vi "ep_Parameter Calculation.vi"(7 "reset? (F)":bool, 8 "error in (no error)":errorcluster, 9 "filter for frequency measurement":T2={"enable filter? (T)"=TRUE, "passband edge frequency [Hz]"=0.0, "passband ripple [dB]"=0.1, "stopband edge frequency [Hz]"=0.0, "stopband attenuation [dB]"=60.0}, 10 "frequency range [Hz]":cluster{"minimum":dbl, "maximum":dbl}, 11 "reference signal":waveform(dbl)) -> (0 "error out":errorcluster, 1 "total group delay [s]":dbl, 2 "parameters":T1, 3 "data out":dbl[](array[numeric]))   [LabVIEW 2013, in "NI_EP_Power Measurement.lvlib"]
uses:
  <vilib>/addons/Electrical Power/Power Measurement/NI_EP_Power Measurement.lvlib
  <vilib>/addons/Electrical Power/Power Measurement/subVIs/ep_Filter Design.ctl
  <vilib>/addons/Electrical Power/PQ/Resampling/Desktop/subVIs/ep_Parameters.ctl
  <vilib>/addons/Electrical Power/PQ/Resampling/NI_EP_Resample_Host.lvlib
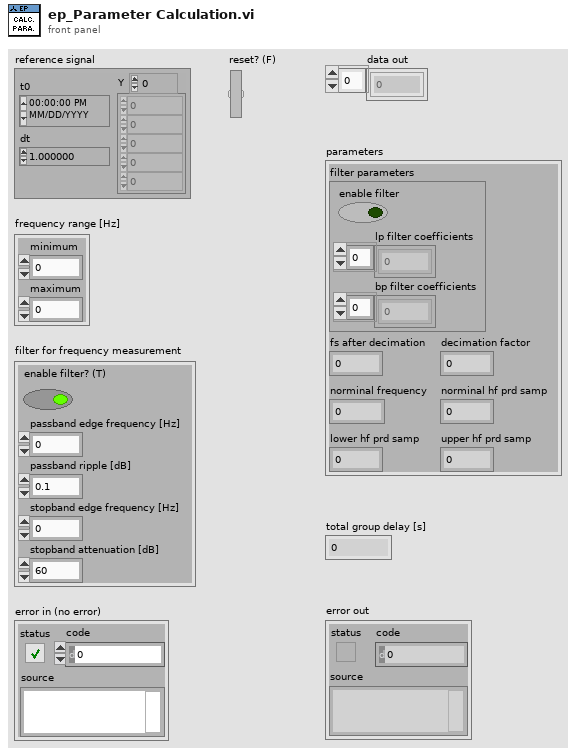
[diagram p1: front panel]
types:
  T1 = typedef "NI_EP_Resample_Host.lvlib/ep_Parameters.ctl" = cluster{"filter parameters":cluster{"enable filter":bool, "lp filter coefficients":dbl[], "bp filter coefficients":dbl[]}, "fs after decimation":dbl, "decimation factor":i32, "norminal frequency":dbl, "norminal hf prd samp":dbl, "lower hf prd samp":i32, "upper hf prd samp":i32}
  T2 = typedef "NI_EP_Power Measurement.lvlib/ep_Filter Design.ctl" = cluster{"enable filter? (T)":bool, "passband edge frequency [Hz]":dbl, "passband ripple [dB]":dbl, "stopband edge frequency [Hz]":dbl, "stopband attenuation [dB]":dbl}
  T3 = cluster{"enable filter":bool, "lp filter coefficients":dbl[], "bp filter coefficients":dbl[]}
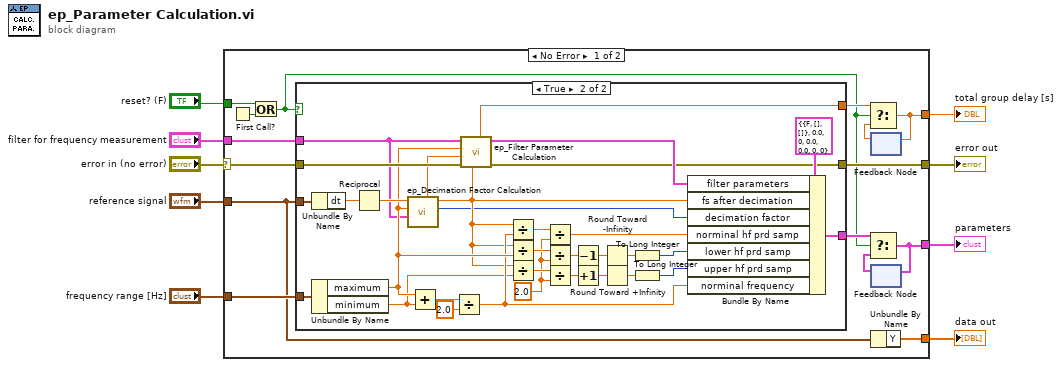
[diagram p0: block diagram]
diagram:
  n1 = case shown="No Error" "error in (no error)" {
    selector: "error in (no error)" -> [w20 w58]
    tunnel: "reset? (F)" -> [w23 _]
    tunnel: "reference signal" -> [w11 _]
    tunnel: "filter for frequency measurement" -> [w22 _]
    tunnel: "frequency range [Hz]" -> [w21 _]
    tunnel: [w19 w58] -> w5
    tunnel: [w16 _] -> w4
    tunnel: [w13 _] -> w3
    tunnel: [w10 _] -> w1
    frame No Error {
      n2 = First Call?() -> (First Call?: T/F=w24:bool)
      n3 = Or(x=w23, y=w24) -> (x .or. y?=w12:bool)
      n4 = case shown="True" w12 {
        tunnel: w11 -> [_ w57]
        tunnel: w22 -> [_ w26]
        tunnel: w21 -> [_ w54]
        tunnel: w20 -> [w25 w50]
        tunnel: [w25 w44] -> w19
        tunnel: [_ w34] -> w15
        tunnel: [_ w45] -> w17
        frame False {
        }
        frame True {
          w35 = 2.0 ("y")
          n5 = Unbundle By Name(w57) -> ("dt"=w56:dbl)
          n6 = Unbundle By Name(w54) -> ("maximum"=w48:dbl, "minimum"=w31:dbl)
          n7 = Reciprocal(x=w56) -> (1/x=w51:dbl)
          n8 = call <vilib>:"ep_Decimation Factor Calculation.vi"("filter for frequency measurement"=w26, "maximum frequency [Hz]"=w48, "fs [Hz]"=w51) -> ("decimation factor"=w28:i32, "fs after decimation [Hz]"=w29:dbl, "dup fs [Hz]"=w30:dbl)  [unwired: 6 in]
          n9 = Add(x=w48, y=w31) -> (x+y=w53:dbl)
          n10 = Divide(x=w53, y=2.0) -> (x/y=w43:dbl)
          n11 = call <vilib>:"ep_Filter Parameter Calculation.vi"("fs after decimation [Hz]"=w29, "error in (no error)"=w50, "fs [Hz]"=w30, "maximum frequency [Hz]"=w48, "filter for frequency measurement"=w26) -> ("error out"=w44:errorcluster, "filter parameters"=w49:T3, "total group delay [s]"=w34:dbl)  [unwired: 4 in]
          n12 = Divide(x=w29, y=w43) -> (x/y=w41:dbl)
          n13 = Divide(x=w29, y=w48) -> (x/y=w40:dbl)
          n14 = Divide(x=w29, y=w31) -> (x/y=w39:dbl)
          n15 = Divide(x=w41, y=w35) -> (x/y=w36:dbl)
          n16 = Divide(x=w40, y=w35) -> (x/y=w37:dbl)
          n17 = Divide(x=w39, y=w35) -> (x/y=w38:dbl)
          n18 = Decrement(x=w37) -> (x-1=w33:dbl)
          n19 = Increment(x=w38) -> (x+1=w32:dbl)
          n20 = Round Toward -Infinity(1:w33) -> (0:w47:dbl)
          n21 = Round Toward +Infinity(x=w32) -> (ceil(x): smallest int >= x=w46:dbl)
          n22 = To Long Integer(number=w47) -> (32bit integer=w42:i32)
          n23 = To Long Integer(number=w46) -> (32bit integer=w27:i32)
          n24 = Bundle By Name(cluster=T1 {"filter parameters"={"enable filter"=FALSE, "lp filter coefficients"=[], "bp filter coefficients"=[]}, "fs after decimation"=0.0, "decimation factor"=0, "norminal frequency"=0.0, "norminal hf prd samp"=0.0, "lower hf prd samp"=0, "upper hf prd samp"=0} ("output cluster 2"), "filter parameters"=w49, "fs after decimation"=w29, "decimation factor"=w28, "norminal hf prd samp"=w36, "lower hf prd samp"=w42, "upper hf prd samp"=w27, "norminal frequency"=w43) -> (w45:T1)
        }
      }
      n25 = feedback #1() -> (w14:dbl)  [unwired: 1 in]
      n26 = Select(t=w15, s=w12, f=w14) -> (s? t:f=w13:dbl)
      n27 = feedback-in #1(w13) -> ()
      n28 = feedback #2() -> (w18:T1)  [unwired: 1 in]
      n29 = Select(t=w17, s=w12, f=w18) -> (s? t:f=w16:T1)
      n30 = feedback-in #2(w16) -> ()
      n31 = Unbundle By Name(w11) -> ("Y"=w10:dbl[])
    }
    frame Error {
    }
  }
  "error out" <- w5
  "parameters" <- w4
  "total group delay [s]" <- w3
  "data out" <- w1
